vi "Angle to Tape.vi"(9 "Distance To Target (ft)":dbl, 10 "Y":dbl, 11 "X":dbl) -> (2 "Polar Plot":picture, 3 "Angle from Robot (deg)":dbl)   [LabVIEW 2013]
uses:
  <vilib>/Utility/miscctls.llb/LVBoundsTypeDef.ctl
panel:
  in  "Plot Color":u32(colorbox)=16715776
  in  "Grid Color":u32(colorbox)
  in  "Visible Section":u16(ring)=4
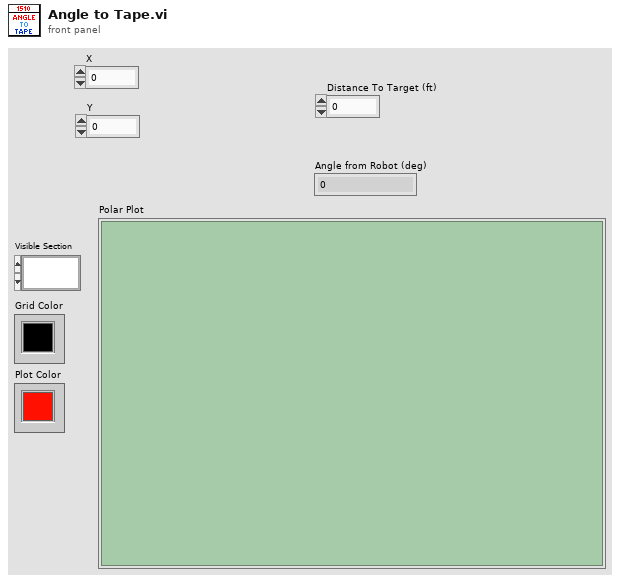
[diagram p1: front panel]
types:
  T1 = typedef "LVBoundsTypeDef.ctl" = cluster{"Width":u32, "Height":u32}
  T2 = cluster{"maximum":dbl, "minimum":dbl, "clip to min":bool, "log?(F)":bool, "grid color":u32, "plot color":u32, "format and precision":cluster{"format":enum8{"Decimal", "Scientific", "Engineering", "Binary", "Octal", "Hex"}, "precision":u8}, "visible section":u16}
  T3 = cluster{"Distance To Target (ft)":dbl, "Radius":dbl}[]
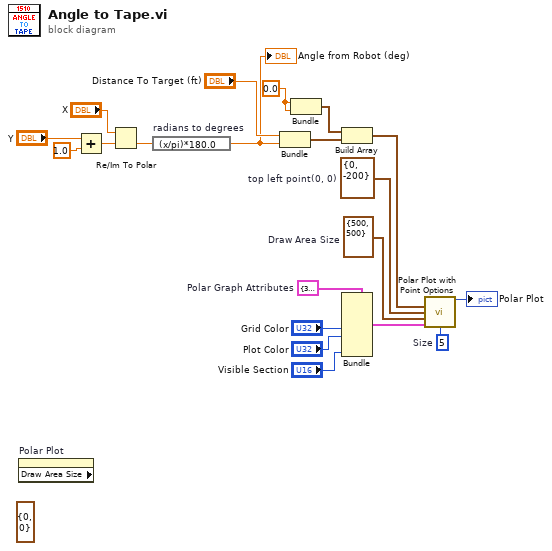
[diagram p0: block diagram]
diagram:
  w1 = T1 {"Width"=500, "Height"=500}  # Draw Area Size
  w2 = cluster{"x":i16, "y":i16} {"x"=0, "y"=-200}  # top left point(0, 0)
  (unwired) T1 {"Width"=0, "Height"=0} ("Draw Area Size")
  w8 = u16 5  # Size
  w9 = 0.0 ("Radius")
  w14 = T2 {"maximum"=30.0, "minimum"=0.0, "clip to min"=FALSE, "log?(F)"=FALSE, "grid color"=6710886, "plot color"=65280, "format and precision"={"format"=enum."Decimal", "precision"=1}, "visible section"=0}  # Polar Graph Attributes
  n1 = property on="Polar Plot" class="Pict" props=["Draw Area Size"]() -> ()  [unwired: 2 in, 3 out]
  n2 = Add(x="Y", y=1.0) -> (x+y=w6:dbl)
  n3 = Re/Im To Polar(2:w6, 3:"X") -> (0:w20:dbl)  [unwired: 1 out]
  n4 = expression code="(x/pi)*180.0" "radians to degrees"(w20) -> (w17:dbl)
  "Angle from Robot (deg)" <- w17
  n5 = Bundle("Distance To Target (ft)"="Distance To Target (ft)", w17) -> (w16:cluster{"Distance To Target (ft)":dbl, dbl})  [unwired: 1 in]
  n6 = Bundle("Radius"=w9, "Radius"=w9) -> (w10:cluster{"Radius":dbl, "Radius":dbl})  [unwired: 1 in]
  n7 = Build Array(w10, w16) -> (w15:T3)
  n8 = Bundle(cluster=w14, "grid color"="Grid Color", "plot color"="Plot Color", "visible section"="Visible Section") -> (w3:T2)  [unwired: 5 in]
  n9 = call <vilib>:"Polar Plot with Point Options.vi"("data array [mag, phase (deg)]"=w15, "top left point(0, 0)"=w2, "dimensions (w,h)"=w1, "polar attributes"=w3, "Size"=w8) -> ("new picture"=→"Polar Plot":picture)  [unwired: 10 in]
